vi "UART_read.vi"(8 "error in":errorcluster, 11 "VISA resource name in":refnum<visa-resource-name>) -> (0 "error out":errorcluster, 2 "UART_out":string, 3 "VISA resource name out":refnum<visa-resource-name>)   [LabVIEW 2025]
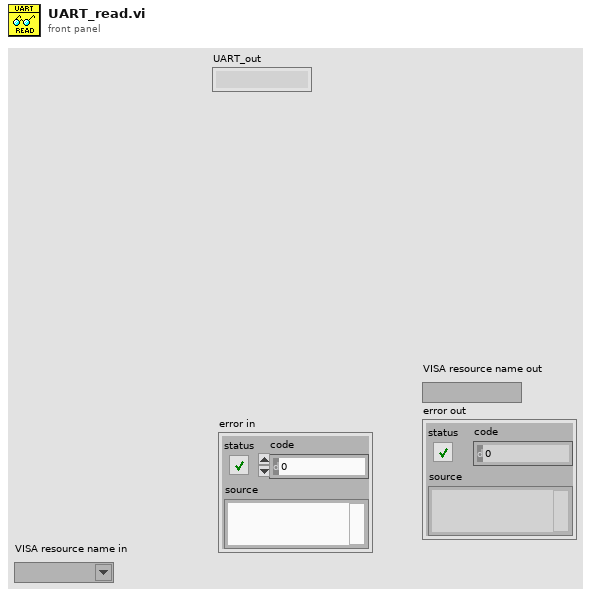
[diagram p1: front panel]
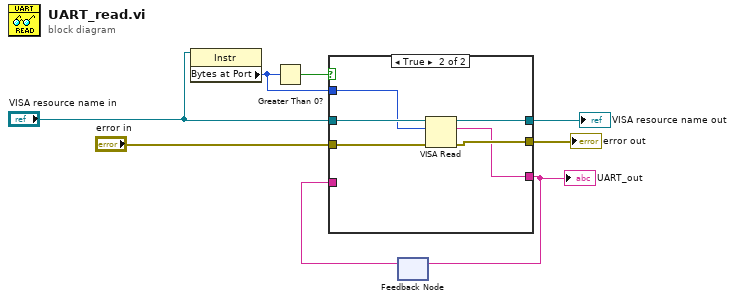
[diagram p0: block diagram]
diagram:
  n1 = property class="Instr"(reference="VISA resource name in") -> ("Bytes at Port"=w7:u32)  [unwired: 1 in, 2 out]
  n2 = Greater Than 0?(x=w7) -> (x > 0?=w8:bool)
  n3 = feedback #1() -> (w3:string)  [unwired: 1 in]
  n4 = case shown="True" w8 {
    tunnel: "error in" -> [w10 w17]
    tunnel: [w11 w16] -> w5
    tunnel: [w10 w15] -> w6
    tunnel: "VISA resource name in" -> [w11 w14]
    tunnel: [w9 w12] -> w4
    tunnel: w7 -> [_ w13]
    tunnel: w3 -> [w9 _]
    frame False {
    }
    frame True {
      n5 = VISA Read(VISA resource name=w14, byte count=w13, error in (no error)=w17) -> (VISA resource name out=w16:refnum<visa-resource-name>, read buffer=w12:string, error out=w15:errorcluster)  [unwired: 1 out]
    }
  }
  "VISA resource name out" <- w5
  "error out" <- w6
  "UART_out" <- w4
  n6 = feedback-in #1(w4) -> ()
